vi "Create_Trajectory_Parse_RectRegion_Constraint.vi"(11 "inTRAJECTORY_CONFIG":T2 {"End Velocity" format="%20.4f"; "StartVelocity" format="%20.4f"; "Max Acceleration" format="%20.4f"; "MaxVelocity" format="%20.4f"}) -> (0 "Constraint Exists":bool, 1 "Max Speed":dbl, 2 "BottomLeftPoint":T1 {"Y" format="%14.3f"; "X" format="%14.3f"}, 3 "TopRightPoint":T1 {"Y" format="%14.3f"; "X" format="%14.3f"})   [LabVIEW 2019]
doc: "Retrieves the Differntial Drive Kinematics constraint from the Trajectory Configuration.\n\nNote: If more than once instance of the Differntial Drive Kinematics constraint exists only the first one is returned. (Only one of these should be defined.)\n\nParameters:\n - InTrajectoryConfig -- The trajectory configuration data structure\n\nReturns:\n - Diff Drive Kinematics Constraint -- The data cluster, which contains the constraint.\n - Constraint Exists -- Returns TRUE if this constraint is defined in the trjaectory configuration."
uses:
  <vilib>/Rock Robotics/WPI/ThirdParty/JAS_Junk/TrajLib/TypeDef/TRAJ_CONSTRAINT_MAX_VELOCITY.ctl
  <vilib>/Rock Robotics/WPI/ThirdParty/JAS_Junk/TrajLib/Trajectory_Library.lvlib
  <vilib>/Rock Robotics/WPI/ThirdParty/JAS_Junk/TrajLib/TypeDef/TRAJ_CONFIG.ctl
  <vilib>/Rock Robotics/WPI/ThirdParty/JAS_Junk/TrajLib/TypeDef/TRANSLATION2D.ctl
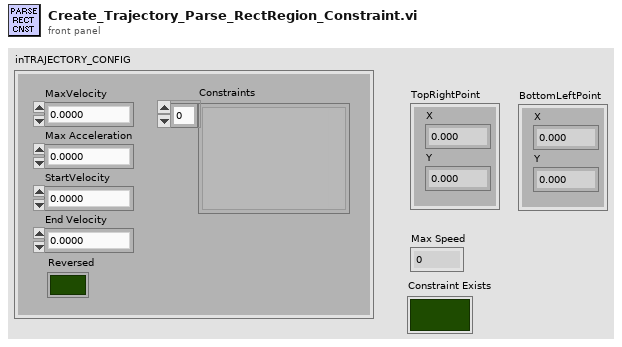
[diagram p1: front panel]
types:
  T1 = typedef "Trajectory_Library.lvlib/TRANSLATION2D.ctl" = cluster{"X":dbl, "Y":dbl}
  T2 = typedef "Trajectory_Library.lvlib/TRAJ_CONFIG.ctl" = cluster{"MaxVelocity":dbl, "Max Acceleration":dbl, "StartVelocity":dbl, "End Velocity":dbl, "Reversed":bool, "Constraints":variant[]}
  T3 = typedef "Trajectory_Library.lvlib/TRAJ_CONSTRAINT_RECT_REGION.ctl" = cluster{"BottomLeftPoint":T1, "TopRightPoint":T1, "Constraint":variant, "Constraint Type":T4}
  T4 = typedef "Trajectory_Library.lvlib/TRAJ_CONSTRAINT_TYPES_ENUM.ctl" = enum16{"UNDEFINED", "DIFF DRIVE KINEMATICS", "DIFF DRIVE VOLTAGE", "CENTRIPITAL ACCEL", "MECA DRIVE KINEMATICS", "SWERVE DRIVE KINEMATICS", "MAXIMUM VELOCITY", "ELLIPTICAL REGION", "RECTANGULAR REGION"}
  T5 = typedef "Trajectory_Library.lvlib/TRAJ_CONSTRAINT_MAX_VELOCITY.ctl" = cluster{"Max Velocity":dbl, "IM UNIQUE":bool}
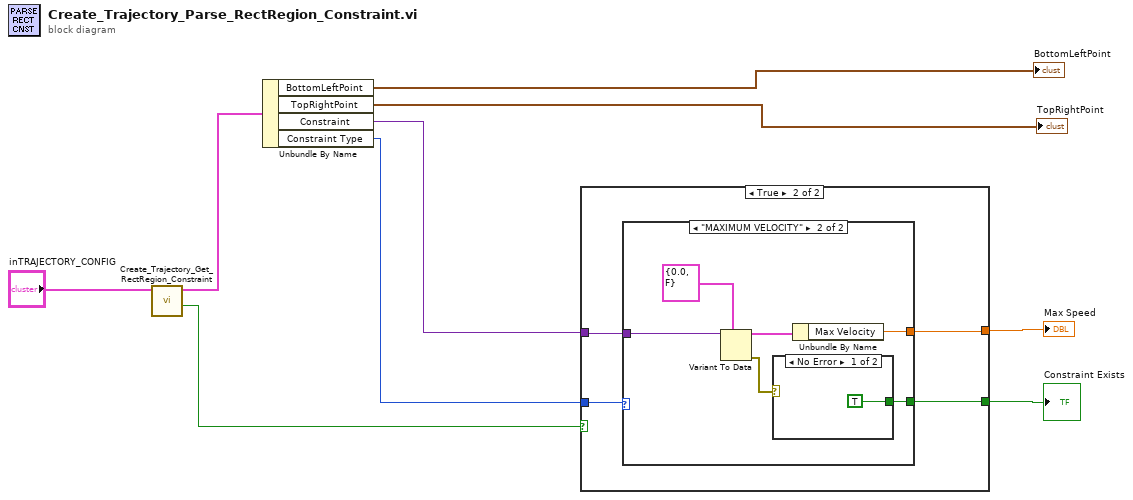
[diagram p0: block diagram]
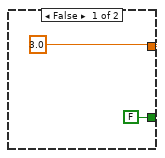
[diagram p2: hidden frame]
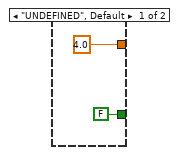
[diagram p3: hidden frame]
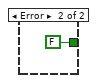
[diagram p4: hidden frame]
diagram:
  n1 = call "Create_Trajectory_Get_RectRegion_Constraint.vi"("inTRAJECTORY_CONFIG"="inTRAJECTORY_CONFIG") -> ("Constraint Exists"=w8:bool, "Rect Region Constraint"=w7:T3)  [unwired: 9 in]
  n2 = Unbundle By Name(w7) -> ("BottomLeftPoint"=→"BottomLeftPoint":T1, "TopRightPoint"=→"TopRightPoint":T1, "Constraint"=w3:variant, "Constraint Type"=w4:T4)
  n3 = case shown="True" w8 {
    tunnel: w4 -> [_ w15]
    tunnel: w3 -> [_ w14]
    tunnel: [3.0 w13] -> w2
    tunnel: [FALSE w12] -> w1
    frame False {
    }
    frame True {
      n4 = case shown="\"MAXIMUM VELOCITY\"" w15 {
        tunnel: w14 -> [_ w23]
        tunnel: [4.0 ("Max Velocity") w20] -> w13
        tunnel: [FALSE w18] -> w12
        frame "UNDEFINED", Default {
        }
        frame "MAXIMUM VELOCITY" {
          n5 = Variant To Data(type=T5 {"Max Velocity"=0.0, "IM UNIQUE"=FALSE} ("MAX_VELOCITY_CONSTRAINT"), Variant=w23) -> (data=w21:T5, error out=w19:errorcluster)  [unwired: 1 in]
          n6 = case shown="No Error" w19 {
            tunnel: [TRUE FALSE] -> w18
            frame No Error {
            }
            frame Error {
            }
          }
          n7 = Unbundle By Name(w21) -> ("Max Velocity"=w20:dbl)
        }
      }
    }
  }
  "Constraint Exists" <- w1
  "Max Speed" <- w2
